vi "Read Data.vi"(6 "chip select  (1st chip)":enum16{"1st chip", "2nd chip"}(ring), 8 "error in (no error)":errorcluster, 11 "HD44780 in":refnum<class "HD44780.lvclass">) -> (0 "error out":errorcluster, 1 "data":u8=97 format="%.0x", 3 "HD44780 out":refnum<class "HD44780.lvclass">)   [LabVIEW 2017, in "HD44780.lvclass"]
uses:
  HD44780.lvclass
  HD44780.lvclass/HD44780.ctl
  Common/HD44780 Common.lvlib
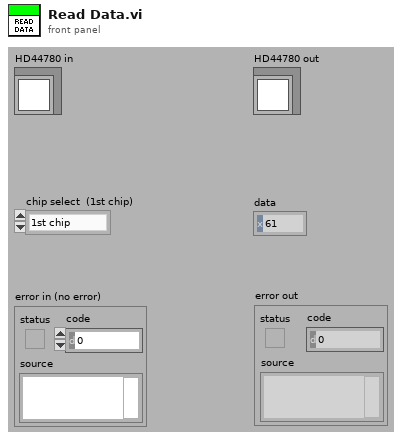
[diagram p1: front panel]
types:
  T1 = typedef "HD44780 Common.lvlib/cluster of class private data.ctl" = cluster{"FPGA VI Reference":refnum<k20>, "device index":i8, "screen size":T2, "font size":T3, "auto wrap":bool, "alignment":T4, "number of line":T5, "shift 0":i8, "entry mode 0":T6, "shift 1":i8, "entry mode 1":T6}
  T2 = typedef "HD44780 Common.lvlib/screen size.ctl" = enum8{"8x1", "8x2", "12x4", "16x1", "16x2", "16x4", "20x1", "20x2", "20x4", "24x1", "24x2", "40x2", "40x4"}
  T3 = typedef "HD44780 Common.lvlib/font size.ctl" = enum8{"5x8", "5x10"}
  T4 = typedef "HD44780 Common.lvlib/alignment.ctl" = enum16{"None", "Left", "Center", "Right"}
  T5 = typedef "HD44780 Common.lvlib/line number.ctl" = enum8{"1 line", "2 lines"}
  T6 = typedef "HD44780 Common.lvlib/entry mode.ctl" = enum8{"increment & no shift", "increment & shift", "decrement & no shift", "decrement & shift"}
  T7 = cluster{"FPGA VI Reference":refnum<k20>, "device index":i8, "screen size":enum8{"8x1", "8x2", "12x4", "16x1", "16x2", "16x4", "20x1", "20x2", "20x4", "24x1", "24x2", "40x2", "40x4"}, "font size":enum8{"5x8", "5x10"}, "auto wrap":bool, "alignment":enum16{"None", "Left", "Center", "Right"}, "number of line":enum8{"1 line", "2 lines"}, "shift 0":i8, "entry mode 0":enum8{"increment & no shift", "increment & shift", "decrement & no shift", "decrement & shift"}, "shift 1":i8, "entry mode 1":enum8{"increment & no shift", "increment & shift", "decrement & no shift", "decrement & shift"}}
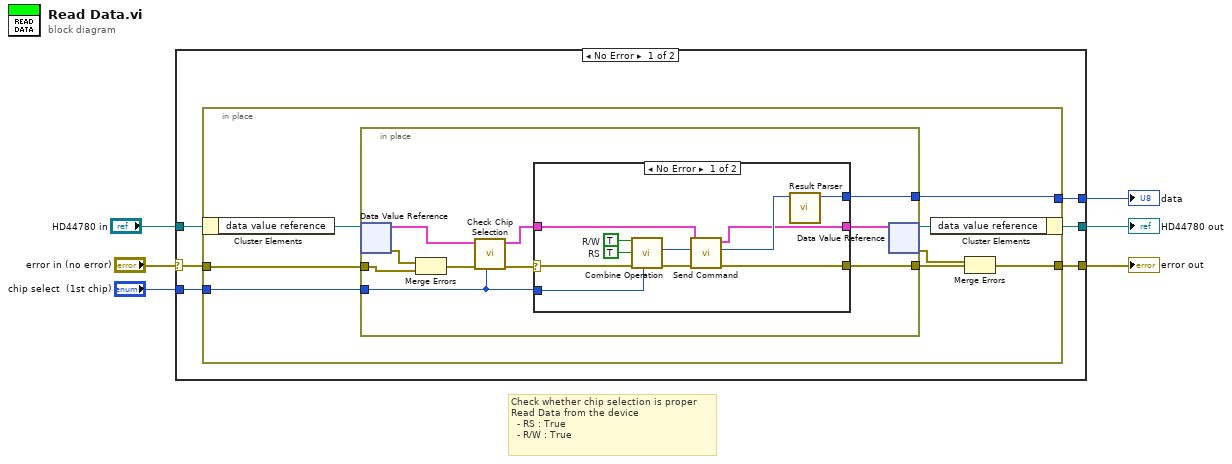
[diagram p0: block diagram]
diagram:
  # "Check whether chip selection is proper\nRead Data from the device\n  - RS : True\n  - R/W : True"
  n1 = case shown="No Error" "error in (no error)" {
    selector: "error in (no error)" -> [w9 w45]
    tunnel: [w12 w45] -> w6
    tunnel: [w11 _] -> w5
    tunnel: "chip select  (1st chip)" -> [w10 _]
    tunnel: "HD44780 in" -> [w8 w44]
    tunnel: [w7 w44] -> w1
    frame No Error {
      n2 = in-place {
        in-place-border: [w20] -> w12
        in-place-border: [w19] -> w11
        in-place-border: w10 -> [w18]
        in-place-border: w9 -> [w17]
        n3 = in-place-cluster #1(w8) -> ("data value reference"=w14:refnum<data-value>)
        n4 = in-place {
          in-place-border: [w30] -> w16
          in-place-border: [w29] -> w19
          in-place-border: w18 -> [w25]
          in-place-border: w17 -> [w27]
          n5 = in-place-dvr #2(w14) -> (w21:T1, w28:errorcluster)
          n6 = Merge Errors(w28, w27) -> (w24:errorcluster)
          n7 = call "Check Chip Selection.vi"("chip select"=w25, "error in (no error)"=w24, "cluster of private data in"=w21) -> ("error out"=w23:errorcluster, "cluster of private data out"=w22:T7)  [unwired: 7 in]
          n8 = case shown="No Error" w23 {
            selector: w23 -> [w38 w43]
            tunnel: [w37 w43] -> w30
            tunnel: [w36 _] -> w29
            tunnel: w25 -> [w31 _]
            tunnel: w22 -> [w32 w42]
            tunnel: [w33 w42] -> w26
            frame No Error {
              w34 = TRUE  # RS
              w41 = TRUE  # R/W
              n9 = call "Combine Operation.vi"("chip select  (1st chip)"=w31, "error in (no error)"=w38, "RS"=w34, "R/W"=w41) -> ("error out"=w40:errorcluster, "output"=w35:u32)  [unwired: 6 in]
              n10 = call "Send Command.vi"("error in (no error)"=w40, "operation"=w35, "cluster of private data in"=w32) -> ("error out"=w37:errorcluster, "result"=w39:u32, "cluster of private data out"=w33:T7)  [unwired: 6 in]
              n11 = call "Result Parser.vi"("operation"=w39) -> ("data"=w36:u8)  [unwired: 8 in, 2 out]
            }
            frame Error {
            }
          }
          n12 = in-place-dvr #2(w26) -> (w13:refnum<data-value>, w15:errorcluster)
        }
        n13 = in-place-cluster #1("data value reference"=w13) -> (w7:refnum<class "HD44780.lvclass">)
        n14 = Merge Errors(w15, w16) -> (w20:errorcluster)
      }
    }
    frame Error {
    }
  }
  "error out" <- w6
  "data" <- w5
  "HD44780 out" <- w1
